vi "Power Fit Coefficients.vi"(0 "Y":dbl[](array[numeric]), 5 "X":dbl[](array[numeric]), 7 "Weight":dbl[](array[numeric]), 9 "tolerance":dbl=0.0001 format="%#_3g", 11 "method":T1 items=["Least Square", "Least Absolute Residual", "Bisquare"]) -> (4 "amplitude":dbl, 6 "power":dbl, 15 "error":i32)   [LabVIEW 2020, in "NI_AALPro.lvlib"]
doc: "Returns the <B>amplitude</B> and <B>power</B> of the power fit for a data set (<B>X</B>, <B>Y</B>) using the Least Square, Least Absolute Residual, or Bisquare method."
uses:
  NI_AALPro.lvlib
  Curve Fitting Criteria.ctl
panel:
  # "Power Fit Coefficients"
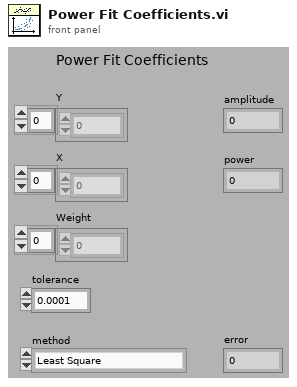
[diagram p1: front panel]
types:
  T1 = typedef "NI_AALPro.lvlib/Curve Fitting Criteria.ctl" = u16
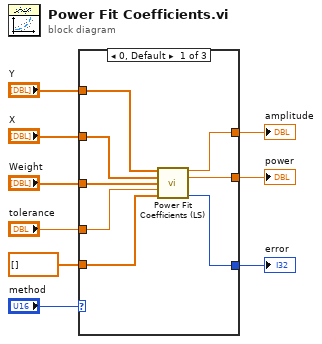
[diagram p0: block diagram]
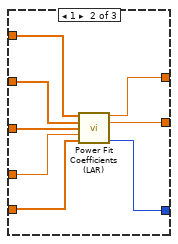
[diagram p2: hidden frame]
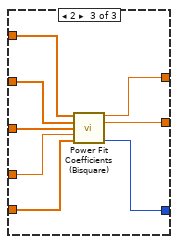
[diagram p3: hidden frame]
diagram:
  n1 = case shown="0, Default" "method" {
    tunnel: "Y" -> [w17 w25 w33]
    tunnel: "X" -> [w16 w24 w32]
    tunnel: "Weight" -> [w15 w23 w31]
    tunnel: "tolerance" -> [w14 w22 w30]
    tunnel: dbl[] [] ("Initial Coefficients") -> [w13 w21 w29]
    tunnel: [w12 w20 w28] -> w3
    tunnel: [w11 w19 w27] -> w2
    tunnel: [w10 w18 w26] -> w1
    frame 0, Default {
      n2 = call "Power Fit Coefficients (LS).vi"("Y"=w17, "X"=w16, "Weight"=w15, "tolerance"=w14, "Initial Coefficients"=w13) -> ("amplitude"=w12:dbl, "power"=w11:dbl, "error"=w10:i32)  [unwired: 8 out]
    }
    frame 1 {
      n3 = call "Power Fit Coefficients (LAR).vi"("Y"=w25, "X"=w24, "Weight"=w23, "tolerance"=w22, "Initial Coefficients"=w21) -> ("amplitude"=w20:dbl, "power"=w19:dbl, "error"=w18:i32)  [unwired: 8 out]
    }
    frame 2 {
      n4 = call "Power Fit Coefficients (Bisquare).vi"("Y"=w33, "X"=w32, "Weight"=w31, "tolerance"=w30, "Initial Coefficients"=w29) -> ("amplitude"=w28:dbl, "power"=w27:dbl, "error"=w26:i32)  [unwired: 8 out]
    }
  }
  "amplitude" <- w3
  "power" <- w2
  "error" <- w1
